vi "convert page nums.vi"(8 "set Card Type":string, 9 "set channel":i32, 10 "set slot":i32, 11 "Cluster":T1) -> (0 "set page":i32, 1 "num pages":i32)   [LabVIEW 2018]
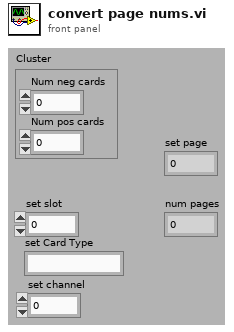
[diagram p1: front panel]
types:
  T1 = cluster{"Num neg cards":i32, "Num pos cards":i32}
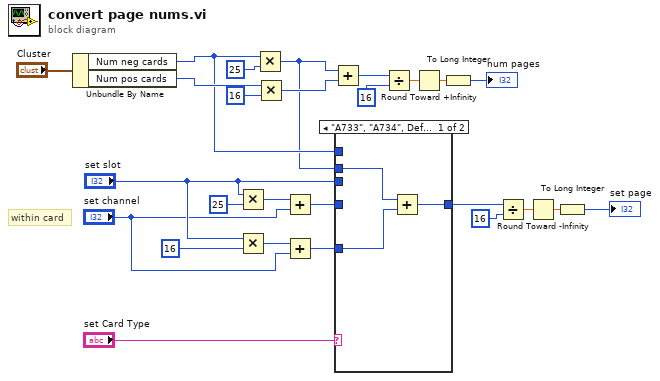
[diagram p0: block diagram]
diagram:
  # "within card"
  n1 = Unbundle By Name("Cluster") -> ("Num neg cards"=w13:i32, "Num pos cards"=w14:i32)
  n2 = Multiply(x="set slot", y=25) -> (x*y=w26:i32)
  n3 = Multiply(x="set slot", y=16) -> (x*y=w11:i32)
  n4 = Multiply(x=w13, y=25) -> (x*y=w8:i32)
  n5 = Multiply(x=w14, y=16) -> (x*y=w24:i32)
  n6 = Add(x=w26, y="set channel") -> (x+y=w1:i32)
  n7 = Add(x=w11, y="set channel") -> (x+y=w7:i32)
  n8 = Add(x=w8, y=w24) -> (x+y=w16:i32)
  n9 = case shown="\"A733\", \"A734\", Default" "set Card Type" {
    tunnel: [w28 w30] -> w3
    tunnel: "set slot" -> [_ _]
    tunnel: w1 -> [_ w30]
    tunnel: w13 -> [_ _]
    tunnel: w8 -> [w29 _]
    tunnel: w7 -> [w27 _]
    frame "A733", "A734", Default {
      n10 = Add(x=w29, y=w27) -> (x+y=w28:i32)
    }
    frame "A938A" {
    }
  }
  n11 = Divide(x=w16, y=16) -> (x/y=w18:dbl)
  n12 = Round Toward +Infinity(x=w18) -> (ceil(x): smallest int >= x=w19:dbl)
  n13 = To Long Integer(number=w19) -> (32bit integer=→"num pages":i32)
  n14 = Divide(x=w3, y=16) -> (x/y=w6:dbl)
  n15 = Round Toward -Infinity(1:w6) -> (0:w5:dbl)
  n16 = To Long Integer(number=w5) -> (32bit integer=→"set page":i32)
